vi "Calculator.vi"() -> ()   [LabVIEW 2020]
panel:
  out "String":string
  in  "Stop":bool
  in  "Cluster":T1
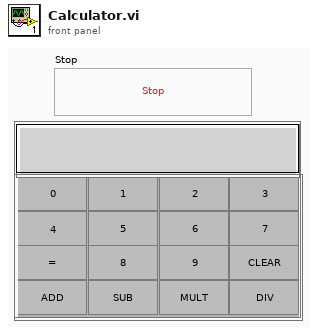
[diagram p1: front panel]
types:
  T1 = cluster{"1":bool, "2":bool, "3":bool, "0":bool, "4":bool, "5":bool, "6":bool, "7":bool, "8":bool, "9":bool, "SUB":bool, "MULT":bool, "DIV":bool, "EQU":bool, "CLEAR":bool, "ADD":bool}
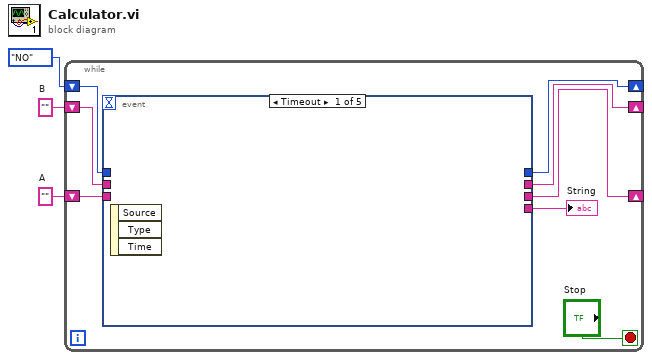
[diagram p0: block diagram]
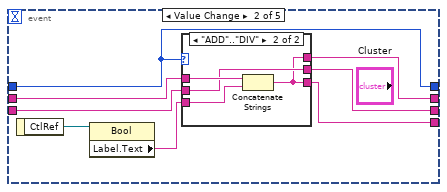
[diagram p2: hidden frame]
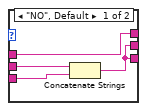
[diagram p3: hidden frame]
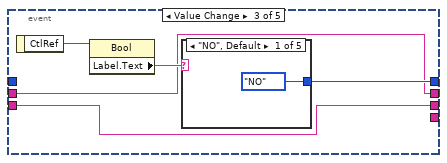
[diagram p4: hidden frame]
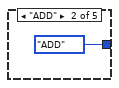
[diagram p5: hidden frame]
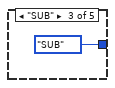
[diagram p6: hidden frame]
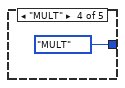
[diagram p7: hidden frame]
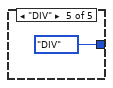
[diagram p8: hidden frame]
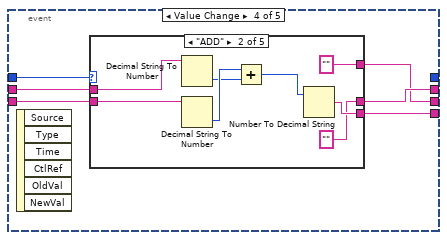
[diagram p9: hidden frame]
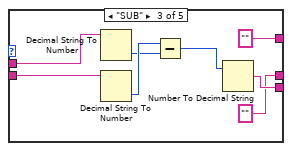
[diagram p11: hidden frame]
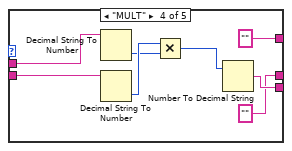
[diagram p12: hidden frame]
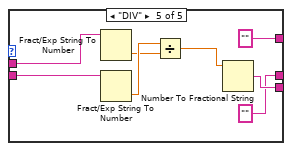
[diagram p13: hidden frame]
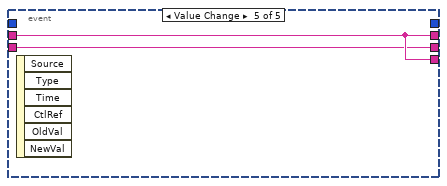
[diagram p14: hidden frame]
diagram:
  w1 = ""  # B
  w2 = ""  # A
  n1 = while {
    shift-right: [w6] -> _
    shift-left: w1 -> [w10]
    shift-right: [w5] -> _
    shift-left: w2 -> [w9]
    shift-right: [w7] -> _
    shift-left: enum16{"NO", "ADD", "SUB", "MULT", "DIV", ""}."NO" -> [w8]
    stop <- "Stop" stop-if-true
    n2 = event shown="[0] Timeout" {
      selector: _ -> [_ _ _ _ _]
      dyn-events: _ -> [_ _ _ _ _]
      timeout: _ -> [_ _ _ _ _]
      tunnel: w10 -> [_ w17 w29 w39 w79]
      tunnel: w9 -> [_ w18 w28 w38 w78]
      tunnel: w8 -> [_ w16 _ w43 _]
      tunnel: [_ w16 w30 _ _] -> w7
      tunnel: [_ w15 w29 w42 w79] -> w6
      tunnel: [_ w14 w28 w41 w78] -> w5
      tunnel: [_ w13 _ w40 w79] -> w4
      event Timeout {
        n3 = event-data() -> ()  [unwired: 1 in, 3 out]
      }
      event "Cluster.0", "Cluster.1", "Cluster.2", "Cluster.3", "Cluster.4", "Cluster.5", "Cluster.6", "Cluster.7", "Cluster.8", "Cluster.9": Value Change {
        n4 = event-data() -> ("CtlRef"=w19:refnum<vi>)  [unwired: 1 in]
        n5 = property class="Bool"(reference=w19) -> ("Label.Text"=w12:string)  [unwired: 1 in, 2 out]
        n6 = case shown="\"ADD\"..\"DIV\"" w16 {
          tunnel: w18 -> [w21 w25]
          tunnel: w17 -> [w22 w26]
          tunnel: [w22 w24] -> w15
          tunnel: [w20 w25] -> w14
          tunnel: [w20 w24] -> w13
          tunnel: w12 -> [w23 w27]
          frame "NO", Default {
            n7 = Concatenate Strings(w21, w23) -> (w20:string)
          }
          frame "ADD".."DIV" {
            n8 = Concatenate Strings(w26, w27) -> (w24:string)
          }
        }
      }
      event "Cluster.ADD", "Cluster.SUB", "Cluster.MULT", "Cluster.DIV": Value Change {
        n9 = event-data() -> ("CtlRef"=w32:refnum<vi>)  [unwired: 1 in]
        n10 = property class="Bool"(reference=w32) -> ("Label.Text"=w31:string)  [unwired: 1 in, 2 out]
        n11 = case shown="\"NO\", Default" w31 {
          tunnel: [enum16{"NO", "ADD", "SUB", "MULT", "DIV", ""}."NO" enum16{"NO", "ADD", "SUB", "MULT", "DIV", ""}."ADD" enum16{"NO", "ADD", "SUB", "MULT", "DIV", ""}."SUB" enum16{"NO", "ADD", "SUB", "MULT", "DIV", ""}."MULT" enum16{"NO", "ADD", "SUB", "MULT", "DIV", ""}."DIV"] -> w30
          frame "NO", Default {
          }
          frame "ADD" {
          }
          frame "SUB" {
          }
          frame "MULT" {
          }
          frame "DIV" {
          }
        }
      }
      event "Cluster.EQU": Value Change {
        n12 = event-data() -> ()  [unwired: 1 in, 6 out]
        n13 = case shown="\"ADD\"" w43 {
          tunnel: [w44 "" "" "" ""] -> w42
          tunnel: w38 -> [w44 w53 w61 w69 w77]
          tunnel: w39 -> [w45 w52 w60 w68 w76]
          tunnel: [w45 "" "" "" ""] -> w41
          tunnel: [w44 w48 w56 w64 w72] -> w40
          frame "NO", Default {
          }
          frame "ADD" {
            n14 = Decimal String To Number(string=w52) -> (number=w50:i32)  [unwired: 2 in, 1 out]
            n15 = Decimal String To Number(string=w53) -> (number=w51:i32)  [unwired: 2 in, 1 out]
            n16 = Add(x=w51, y=w50) -> (x+y=w49:i32)
            n17 = Number To Decimal String(number=w49) -> (decimal integer string=w48:string)  [unwired: 1 in]
          }
          frame "SUB" {
            n18 = Decimal String To Number(string=w60) -> (number=w58:i32)  [unwired: 2 in, 1 out]
            n19 = Decimal String To Number(string=w61) -> (number=w59:i32)  [unwired: 2 in, 1 out]
            n20 = Subtract(x=w59, y=w58) -> (x-y=w57:i32)
            n21 = Number To Decimal String(number=w57) -> (decimal integer string=w56:string)  [unwired: 1 in]
          }
          frame "MULT" {
            n22 = Decimal String To Number(string=w68) -> (number=w66:i32)  [unwired: 2 in, 1 out]
            n23 = Decimal String To Number(string=w69) -> (number=w67:i32)  [unwired: 2 in, 1 out]
            n24 = Multiply(x=w67, y=w66) -> (x*y=w65:i32)
            n25 = Number To Decimal String(number=w65) -> (decimal integer string=w64:string)  [unwired: 1 in]
          }
          frame "DIV" {
            n26 = Fract/Exp String To Number(string=w76) -> (number=w74:dbl)  [unwired: 3 in, 1 out]
            n27 = Fract/Exp String To Number(string=w77) -> (number=w75:dbl)  [unwired: 3 in, 1 out]
            n28 = Divide(x=w75, y=w74) -> (x/y=w73:dbl)
            n29 = Number To Fractional String(number=w73) -> (F-format string=w72:string)  [unwired: 3 in]
          }
        }
      }
      event "Cluster.CLEAR": Value Change {
        n30 = event-data() -> ()  [unwired: 1 in, 6 out]
      }
    }
    "String" <- w4
  }
